vi "Multiple Connections - Client Tx2.vi"() -> ()   [LabVIEW 2011]
doc: "Establishes a connection to the specified host and port and reads the date and time data sent by the Server. It first reads 4 bytes defining the length of the date & time string and then reads the data. After you click the stop button, this VI sends a single character to tell the Date Server VI to terminate the connection.\n\n<B>Note:</B> Requires the use of the Multiple Connections - Server.vi."
panel:
  in  "data in":string="56789:43210"
  in  "Send":bool
  in  "stop":bool
  in  "Machine":string="localhost"
  in  "Port":u16=6341
  # "Instructions:\n1. Open the Multiple Connections - Server.vi.\n2. Run the Multiple Connections - Server.vi first.\n3. Run the Client VIs second.\n4. Stop this VI and restart it to notice the # of Connections on the Server VI change.\n5. Stop the Server VI.  This VI will stop when it times out."
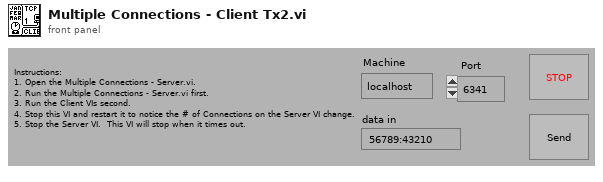
[diagram p1: front panel]
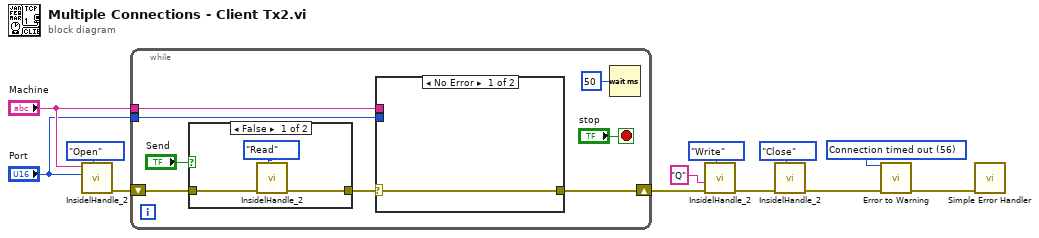
[diagram p0: block diagram]
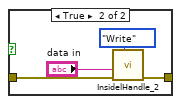
[diagram p2: hidden frame]
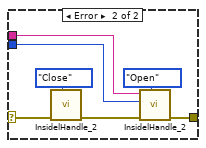
[diagram p3: hidden frame]
diagram:
  w3 = 56 items=["No Error", "Argument Error", "Memory Full", "Out of Zone", "End of File", "File Already Open", "Generic File IO Error", "File Not Found", "File Permission Error", "Disk Full", "Duplicate Path", "Too Many Files Open", "Not Enabled", "Resource File Not Found", "Cannot Add Resource", "Resource Not Found", "Image Not Found", "Image Memory Error", "Pen Does Not Exist", "Config Bad Type", "Config Token Not Found", "Config Parse Error", "Config Memory Error", "Bad External Code Format", "Bad External Code Offset", "External Code Not Present", "Null Window", "Destroy Window Mixup", "Null Menu", "Print Aborted", "Bad Print Record", "Print Driver Error", "Windows Error During Print", "Memory Error During Print", "Print Dialog Error", "Generic Print Error", "Invalid Device Refnum", "Device Not Found", "Device Parameter Error", "Device Unit Error", "Can't Open Device", "Device Call Aborted", "Generic Error", "Cancelled By User", "Object ID Too Low", "Object ID Too High", "Object Not In Heap", "Unknown Heap", "Bad DefProc ID", "DefProc Not In Table", "Message Out Of Range", "Null Method", "Unknown Message", "Manager Call Not Supported", "Bad address", "Connection In progress", "Connection timed out", "Connection is already in progress", "Network attribute not supported", "Network error", "Address in use", "System out of memory", "Connection aborted", "Connection refused", "Connection is not connected", "Connection is already connected", "Connection closed", "Initialize error (interapplication manager)", "Bad occurrence", "Wait on unbound occurrence handler", "Occurrence queue overflow", "Bad path", "Semaphore not signaled", "Unrecognized type (interapplication manager)"] ("1st Error to Convert")
  n1 = call "InsidelHandle_2.vi"("Mode"=enum16{"Open", "Read", "Write", "Close"}."Open", "Port"="Port", "Machine"="Machine") -> ("error out"=w11:errorcluster)  [unwired: 7 in, 1 out]
  n2 = while {
    shift-right: [w19] -> w7
    shift-left: w11 -> [w18]
    tunnel: "Machine" -> [w16]
    tunnel: "Port" -> [w15]
    stop <- "stop" stop-if-true
    n3 = case shown="False" "Send" {
      tunnel: w18 -> [w22 w27]
      tunnel: [w21 w26] -> w17
      frame False {
        n4 = call "InsidelHandle_2.vi"("Mode"=enum16{"Open", "Read", "Write", "Close"}."Read", "error in (no error)"=w22) -> ("error out"=w21:errorcluster)  [unwired: 8 in, 1 out]
      }
      frame True {
        n5 = call "InsidelHandle_2.vi"("Mode"=enum16{"Open", "Read", "Write", "Close"}."Write", "error in (no error)"=w27, "data in"="data in") -> ("error out"=w26:errorcluster)  [unwired: 7 in, 1 out]
      }
    }
    n6 = case shown="No Error" w17 {
      selector: w17 -> [w28 w31]
      tunnel: [w28 w32] -> w19
      tunnel: w16 -> [_ w30]
      tunnel: w15 -> [_ w29]
      frame No Error {
      }
      frame Error {
        n7 = call "InsidelHandle_2.vi"("Mode"=enum16{"Open", "Read", "Write", "Close"}."Close", "error in (no error)"=w31) -> ("error out"=w33:errorcluster)  [unwired: 8 in, 1 out]
        n8 = call "InsidelHandle_2.vi"("Mode"=enum16{"Open", "Read", "Write", "Close"}."Open", "error in (no error)"=w33, "Port"=w29, "Machine"=w30) -> ("error out"=w32:errorcluster)  [unwired: 6 in, 1 out]
      }
    }
    n9 = Wait (ms)(milliseconds to wait=u32 50) -> ()  [unwired: 1 out]
  }
  n10 = call "InsidelHandle_2.vi"("Mode"=enum16{"Open", "Read", "Write", "Close"}."Write", "error in (no error)"=w7, "data in"="Q") -> ("error out"=w8:errorcluster)  [unwired: 7 in, 1 out]
  n11 = call "InsidelHandle_2.vi"("Mode"=enum16{"Open", "Read", "Write", "Close"}."Close", "error in (no error)"=w8) -> ("error out"=w2:errorcluster)  [unwired: 8 in, 1 out]
  n12 = call <vilib>:"Error to Warning.vi"("1st Error to Convert"=w3, "error in"=w2) -> ("warning out"=w1:errorcluster)  [unwired: 3 in, 10 out]
  n13 = call <vilib>:"Simple Error Handler.vi"("error in (no error)"=w1) -> ()  [unwired: 1 in, 8 out]
